vi "TestProgram3multimeter.vi"() -> ()   [LabVIEW 2011]
panel:
  out "Return":string
  in  "Set Temperature Command":string
  in  "Set Temperature":bool
  out "Return Value Temp":string
  in  "Command Temp":string
  in  "Temp":refnum<visa-resource-name>
  out "Return Value 3":string
  out "Return Value 2":string
  out "Return Value 1":string
  in  "Command 3":string
  in  "Command 2":string
  in  "Command  1":string
  in  "Multimeter 3":refnum<visa-resource-name>
  in  "Multimeter 2":refnum<visa-resource-name>
  in  "Multimeter 1":refnum<visa-resource-name>
  in  "Measure":bool
  in  "stop":bool
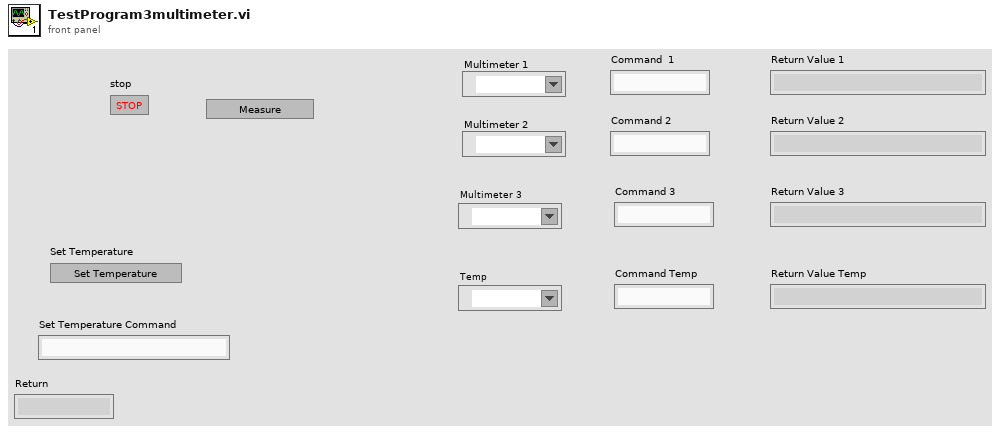
[diagram p1: front panel]
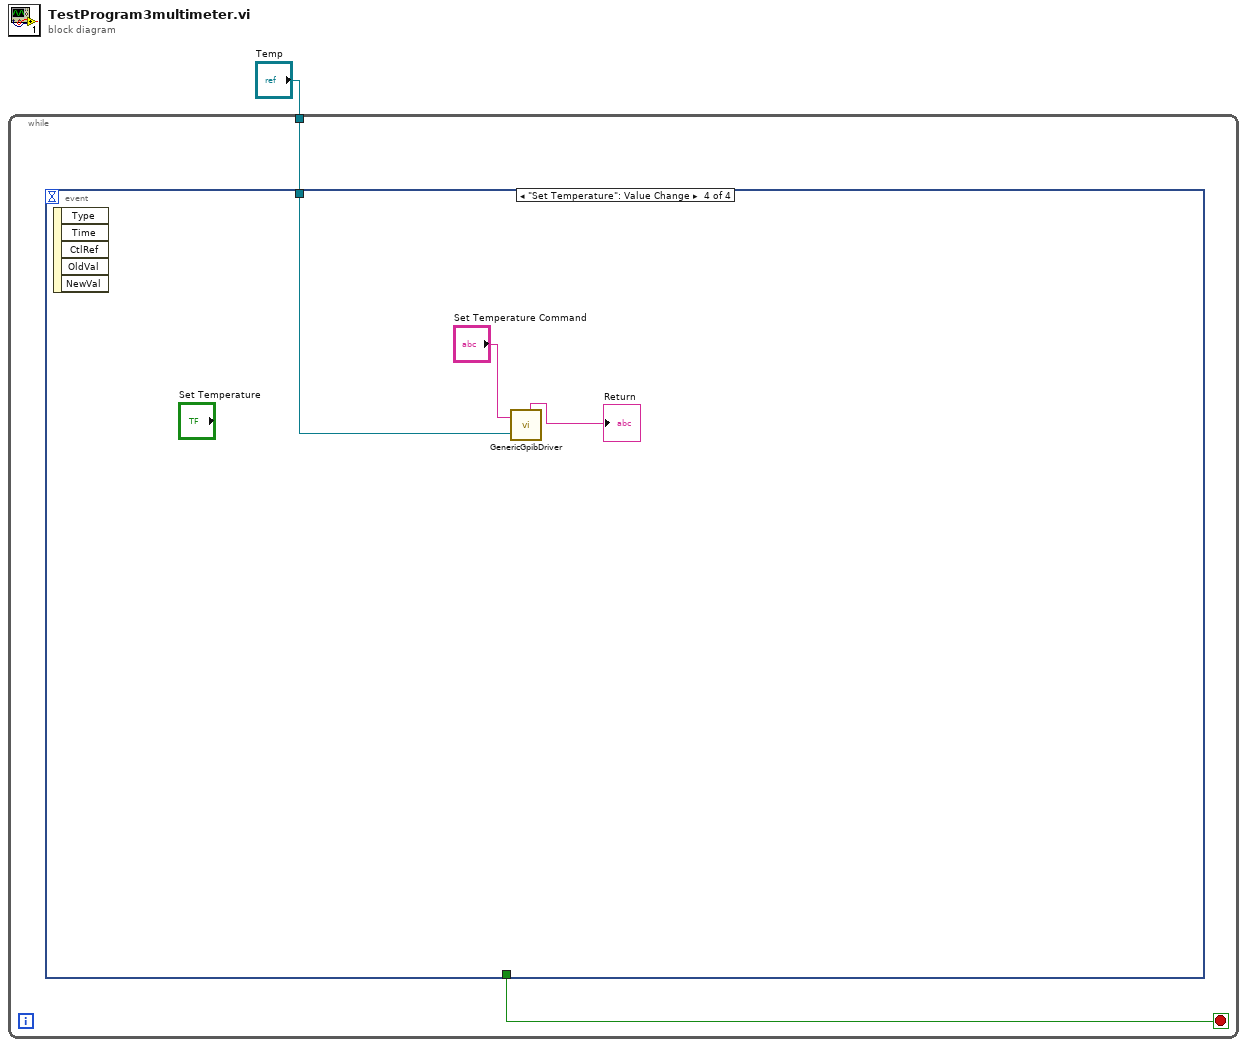
[diagram p0: block diagram]
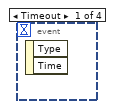
[diagram p2: hidden frame]
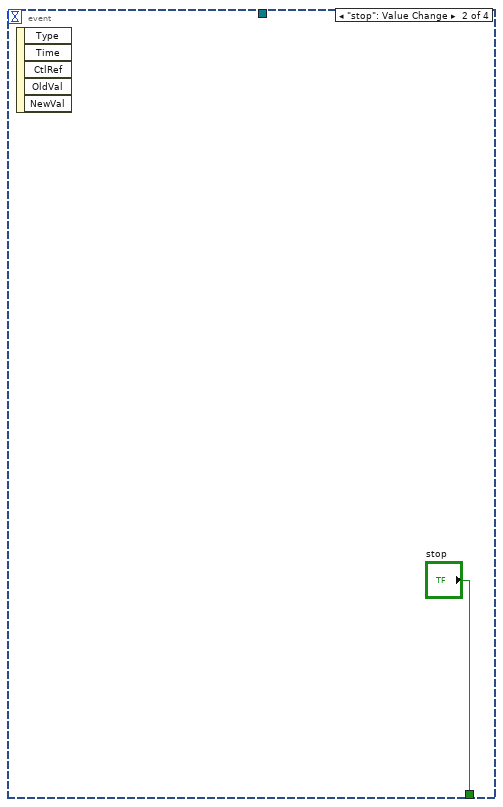
[diagram p3: hidden frame]
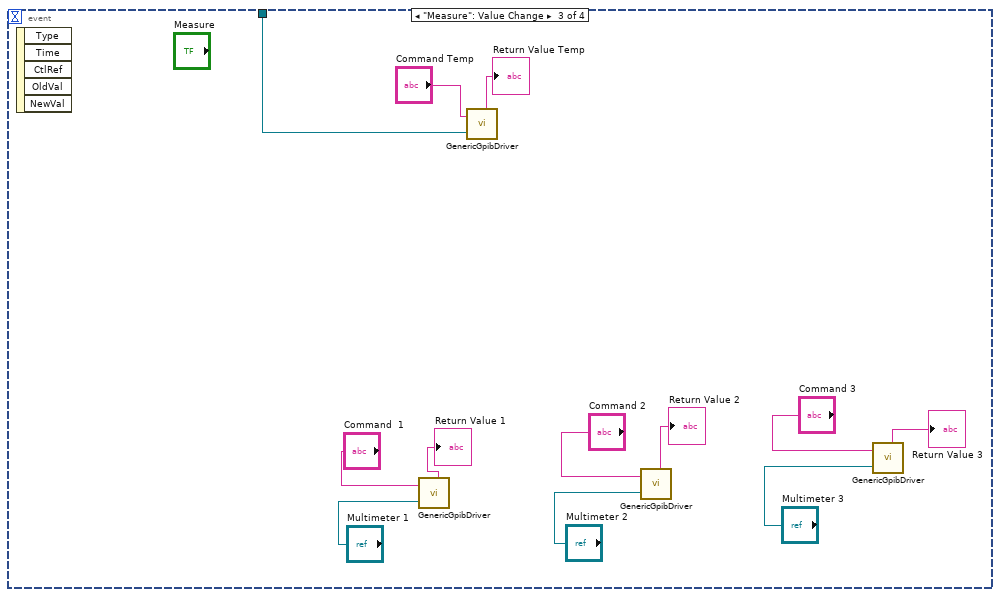
[diagram p4: hidden frame]
diagram:
  n1 = while {
    tunnel: "Temp" -> [w2]
    stop <- w3 stop-if-true
    n2 = event shown="[3] \"Set Temperature\": Value Change" {
      selector: _ -> [_ _ _ _]
      dyn-events: _ -> [_ _ _ _]
      timeout: _ -> [_ _ _ _]
      tunnel: [_ "stop" _ _] -> w3
      tunnel: w2 -> [_ _ w5 w18]
      event Timeout {
        n3 = event-data() -> ()  [unwired: 1 in, 2 out]
      }
      event "stop": Value Change {
        n4 = event-data() -> ()  [unwired: 1 in, 5 out]
      }
      event "Measure": Value Change {
        n5 = event-data() -> ()  [unwired: 1 in, 5 out]
        n6 = call "GenericGpibDriver.vi"("VISA resource name"="Multimeter 1", "Command"="Command  1") -> ("Return Value"=→"Return Value 1":string)  [unwired: 4 out]
        n7 = call "GenericGpibDriver.vi"("VISA resource name"=w5, "Command"="Command Temp") -> ("Return Value"=→"Return Value Temp":string)  [unwired: 4 out]
        n8 = call "GenericGpibDriver.vi"("VISA resource name"="Multimeter 2", "Command"="Command 2") -> ("Return Value"=→"Return Value 2":string)  [unwired: 4 out]
        n9 = call "GenericGpibDriver.vi"("VISA resource name"="Multimeter 3", "Command"="Command 3") -> ("Return Value"=→"Return Value 3":string)  [unwired: 4 out]
      }
      event "Set Temperature": Value Change {
        n10 = event-data() -> ()  [unwired: 1 in, 5 out]
        n11 = call "GenericGpibDriver.vi"("VISA resource name"=w18, "Command"="Set Temperature Command") -> ("Return Value"=→"Return":string)  [unwired: 4 out]
      }
    }
  }
